vi "PCO_GetPlayPositionHDSDI.vi"(8 "error in (no error)":errorcluster {"code" format="%x"}, 11 "ph":u64) -> (0 "error out":errorcluster {"code" format="%x"}, 1 "wStatus":u16(ring) items=["not active", "active"], 2 "ErrorMessage":i32 format="%x", 3 "ph out":u64, 5 "dwPlayPosition":u32)   [LabVIEW 2020, in "SDK.lvlib" / "SpecialCommandsDimax_HDSDI.lvlib"]
doc: "<b>Description:</b>\nThe function PCO_GetPlayPositionHDSDI queries the current position of the play pointer of the currently started sequence. Due to time necessary for communication and processing of the command, the current pointer may be 1 or 2 steps images ahead at the time, when the function returns.\n\n<b>Supported camera type:</b>\npco.dimax with HD-SDI interface\n\n<b>Descriptor dependency:</b>\nNone"
uses:
  SpecialCommandsDimax_HDSDI.lvlib
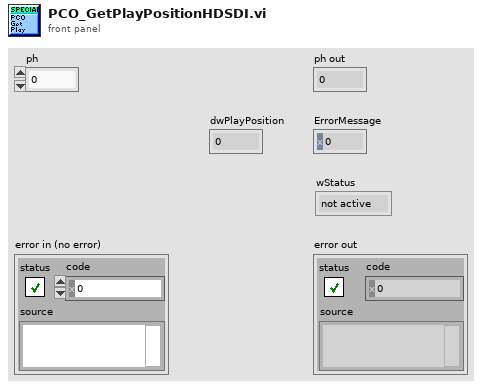
[diagram p1: front panel]
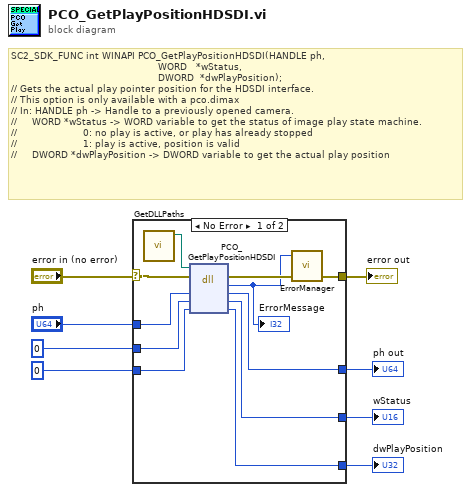
[diagram p0: block diagram]
diagram:
  # "SC2_SDK_FUNC int WINAPI PCO_GetPlayPositionHDSDI(HANDLE ph,\n                                                 WORD   *wStatus,\n                                                 DWORD  *dwPlayPosition);\n// Gets the actual play pointer position for the HDSDI interface.\n// This option is only available with a pco.dimax\n// In: HANDLE ph -> Handle to a previously opened camera.\n//     WORD *wStatus -> WORD variable to get the status of image play state machine.\n//                      0: no play is active, or play has already stopped\n//                      1: play is active, position is valid\n//     DWORD *dwPlayPosition -> DWORD variable to get the actual play position"
  n1 = case shown="No Error" "error in (no error)" {
    selector: "error in (no error)" -> [w13 w23]
    tunnel: "ph" -> [w19 w22]
    tunnel: [w18 w22] -> w7
    tunnel: u16 0 ("wStatus") -> [w17 w21]
    tunnel: [w16 w21] -> w5
    tunnel: u32 0 ("dwPlayPosition") -> [w15 w20]
    tunnel: [w14 w20] -> w3
    tunnel: [w12 w23] -> w2
    frame No Error {
      n2 = call "GetDLLPaths.vi"() -> ("SC2_Cam_Path"=w9:path)  [unwired: 9 in, 2 out]
      n3 = dll-call lib="?" fn="PCO_GetPlayPositionHDSDI"(path in=w9, error in=w13, "ph"=w19, "wStatus"=w17, "dwPlayPosition"=w15) -> (error out=w11:errorcluster, "return type"=w10:i32, "ph"=w18:u64, "wStatus"=w16:u16, "dwPlayPosition"=w14:u32)  [unwired: 1 in, 1 out]
      "ErrorMessage" <- w10
      n4 = call "ErrorManager.vi"("error in (no error)"=w11, "error code"=w10) -> ("error out"=w12:errorcluster)  [unwired: 3 in]
    }
    frame Error {
    }
  }
  "ph out" <- w7
  "wStatus" <- w5
  "dwPlayPosition" <- w3
  "error out" <- w2
